vi "Comments.Add Device Description.vi"(8 "error in (no error)":errorcluster, 11 "Control Experiment in":refnum<class "Control Experiment.lvclass">) -> (0 "error out":errorcluster, 3 "Control Experiment out":refnum<class "Control Experiment.lvclass">)   [LabVIEW 2019, in "Control Experiment.lvclass"]
uses:
  Control Experiment.lvclass
  Control Experiment.lvclass/Control Experiment.ctl
  <userlib>/LevyLab/PLYM/YAML.lvclass
panel:
  out "Device Description":string
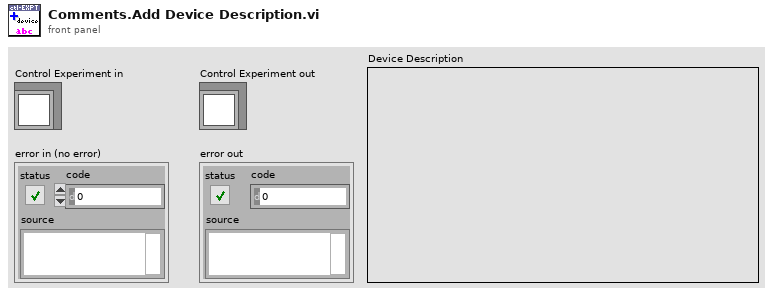
[diagram p1: front panel]
types:
  T1 = typedef "Control Experiment.lvclass/Instrument--enum.ctl" = enum16{"----- AFM/EBL -----", "AGILENT", "CYPHER", "Gemini2", "JEOL", "MFP3D", "----- Cryostat -----", "CF900", "DR200", "MNK", "PPMS (simulated)", "PPMS 1", "PPMS 2", "PPMS 3", "----- Optics -----", "THz 1 (Element 2/Montana)", "THz 2 (Tsunami/Janis)"}
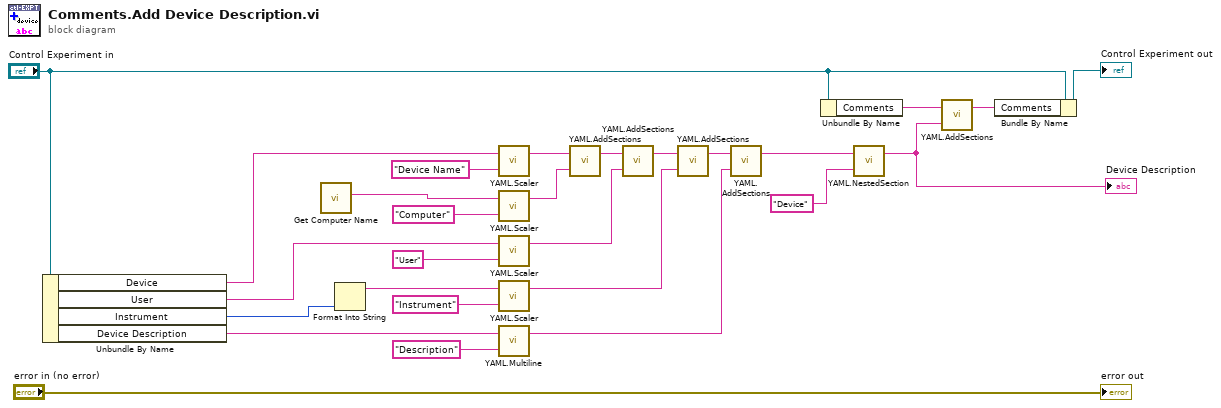
[diagram p0: block diagram]
diagram:
  n1 = Unbundle By Name("Control Experiment in") -> ("Device"=w8:string, "User"=w11:string, "Instrument"=w7:T1, "Device Description"=w16:string)
  n2 = call "Get Computer Name.vi"() -> ("name"=w2:string)  [unwired: 10 in, 1 out]
  n3 = Format Into String(w7) -> (resulting string=w14:string)  [unwired: 3 in, 1 out]
  n4 = call <userlib>:"YAML.Scaler.vi"("Key"="Device Name" ("string"), "Scaler"=w8) -> ("Output"=w25:string)  [unwired: 1 in]
  n5 = call <userlib>:"YAML.Scaler.vi"("Key"="Computer" ("string"), "Scaler"=w2) -> ("Output"=w17:string)  [unwired: 1 in]
  n6 = call <userlib>:"YAML.Scaler.vi"("Key"="User" ("string"), "Scaler"=w11) -> ("Output"=w19:string)  [unwired: 1 in]
  n7 = call <userlib>:"YAML.Scaler.vi"("Key"="Instrument" ("string"), "Scaler"=w14) -> ("Output"=w20:string)  [unwired: 1 in]
  n8 = call <userlib>:"YAML.Multiline.vi"("Key"="Description" ("string"), "Multiline"=w16) -> ("Output"=w21:string)  [unwired: 1 in]
  n9 = call <userlib>:"YAML.AddSections.vi"("Section 2"=w17, "Section 1"=w25) -> ("Output"=w18:string)  [unwired: 1 in]
  n10 = call <userlib>:"YAML.AddSections.vi"("Section 2"=w19, "Section 1"=w18) -> ("Output"=w22:string)  [unwired: 1 in]
  n11 = call <userlib>:"YAML.AddSections.vi"("Section 2"=w20, "Section 1"=w22) -> ("Output"=w23:string)  [unwired: 1 in]
  n12 = call <userlib>:"YAML.AddSections.vi"("Section 2"=w21, "Section 1"=w23) -> ("Output"=w26:string)  [unwired: 1 in]
  n13 = Unbundle By Name("Control Experiment in") -> ("Comments"=w4:string)
  n14 = call <userlib>:"YAML.NestedSection.vi"("Section Key"="Device" ("string"), "Nested Section"=w26) -> ("String"=w3:string)  [unwired: 1 in]
  "Device Description" <- w3
  n15 = call <userlib>:"YAML.AddSections.vi"("Section 2"=w3, "Section 1"=w4) -> ("Output"=w27:string)  [unwired: 1 in]
  n16 = Bundle By Name(cluster="Control Experiment in", "Comments"=w27) -> (→"Control Experiment out":refnum<class "Control Experiment.lvclass">)
  "error out" <- "error in (no error)"
